vi "ReadTargetsConfigurationFile.vi"(8 "error in (no error)":errorcluster, 11 "targets.ini file":path) -> (0 "error out":errorcluster, 3 "Targets Configuration":T1)   [LabVIEW 2027, in "VeriStandTestUtilities.lvlib"]
uses:
  VeriStandTestUtilities.lvlib
  TargetsConfiguration.ctl
  TargetPlatform.ctl
  <vilib>/Utility/config.llb/Read Key (String).vi
  <vilib>/Utility/config.llb/NI_LVConfig.lvlib
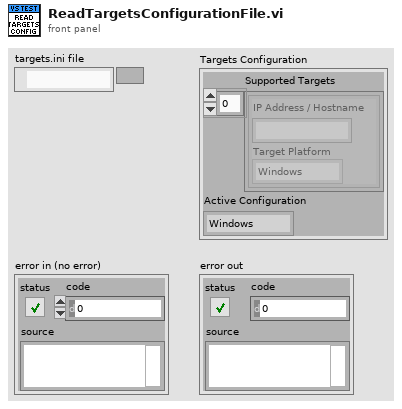
[diagram p1: front panel]
types:
  T1 = typedef "VeriStandTestUtilities.lvlib/TargetsConfiguration.ctl" = cluster{"Supported Targets":cluster{"IP Address / Hostname":string, "Target Platform":T2}[], "Active Configuration":T2}
  T2 = typedef "VeriStandTestUtilities.lvlib/TargetPlatform.ctl" = enum16{"Windows", "Linux64CRIO", "Linux64PXI", "LinuxARM", "PharLap"}
  T3 = cluster{"IP Address / Hostname":string, "Target Platform":T2}
  T4 = typedef "NI_LVConfig.lvlib/Config Data RefNum.ctl" = refnum<k1>
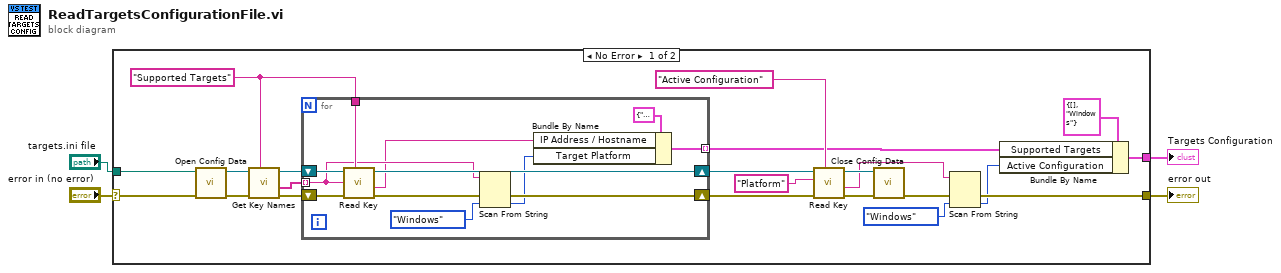
[diagram p0: block diagram]
diagram:
  n1 = case shown="No Error" "error in (no error)" {
    selector: "error in (no error)" -> [w25 w39]
    tunnel: [w7 w39] -> w3
    tunnel: "targets.ini file" -> [w26 _]
    tunnel: [w11 _] -> w1
    frame No Error {
      w22 = "Supported Targets" ("section")
      n2 = call <vilib>:"Open Config Data.vi"("error in (no error)"=w25, "configuration file path"=w26) -> ("error out"=w24:errorcluster, "refnum"=w23:T4)  [unwired: 7 in, 1 out]
      n3 = call <vilib>:"Get Key Names.vi"("section"=w22, "error in (no error)"=w24, "refnum"=w23) -> ("error out"=w21:errorcluster, "key names"=w19:string[], "refnum out"=w20:T4)  [unwired: 5 in, 1 out]
      n4 = for {
        tunnel: w22 -> [w37]
        shift-right: [w29] -> w18
        shift-left: w21 -> [w36]
        shift-right: [w38] -> w17
        shift-left: w20 -> [w35]
        tunnel: w19 -> [w32] mode=indexing
        tunnel: [w34] -> w10 mode=indexing
        n5 = call-poly <vilib>:"Read Key.vi"("section"=w37, "error in (no error)"=w36, "key"=w32, "refnum"=w35) -> ("error out"=w30:errorcluster, "value"=w28:string, "refnum out"=w38:T4)  [unwired: 4 in, 1 out]
        n6 = Scan From String(input string=w32, error in=w30, default 1=TargetPlatform."Windows" ("Active Configuration")) -> (error out=w29:errorcluster, output 1=w27:T2)  [unwired: 2 in, 2 out]
        n7 = Bundle By Name(cluster=T3 {"IP Address / Hostname"="", "Target Platform"=enum."Windows"} ("Target Configuration"), "IP Address / Hostname"=w28, "Target Platform"=w27) -> (w34:T3)
      }
      n8 = call-poly <vilib>:"Read Key.vi"("section"="Active Configuration", "error in (no error)"=w18, "key"="Platform", "refnum"=w17) -> ("error out"=w16:errorcluster, "value"=w6:string, "refnum out"=w15:T4)  [unwired: 4 in, 1 out]
      n9 = call <vilib>:"Close Config Data.vi"("error in (no error)"=w16, "refnum"=w15) -> ("error out"=w8:errorcluster)  [unwired: 8 in, 1 out]
      n10 = Scan From String(input string=w6, error in=w8, default 1=TargetPlatform."Windows" ("Active Configuration")) -> (error out=w7:errorcluster, output 1=w5:T2)  [unwired: 2 in, 2 out]
      n11 = Bundle By Name(cluster=T1 {"Supported Targets"=[], "Active Configuration"=enum."Windows"} ("Targets Configuration"), "Supported Targets"=w10, "Active Configuration"=w5) -> (w11:T1)
    }
    frame Error {
    }
  }
  "Targets Configuration" <- w1
  "error out" <- w3
